vi "file - write list of lines.vi"(7 "read/write control":T1, 10 "list of lines IN":string[](array[string]), 11 "file path":path=path "\\\\rus-one\\newdata/data/Ultrasound/Experiment/ProbeTest/Probe10/Hg1201-6-C185-550Cair-3c-83K/sweep3/9w/3366_a.dat") -> (1 "first line":string, 2 "list of lines OUT":string[](array[string]))   [LabVIEW 2015]
uses:
  file -- read-write control.ctl
  <vilib>/Utility/file.llb/Read From Spreadsheet File (string).vi
  <vilib>/Utility/file.llb/Write To Spreadsheet File (string).vi
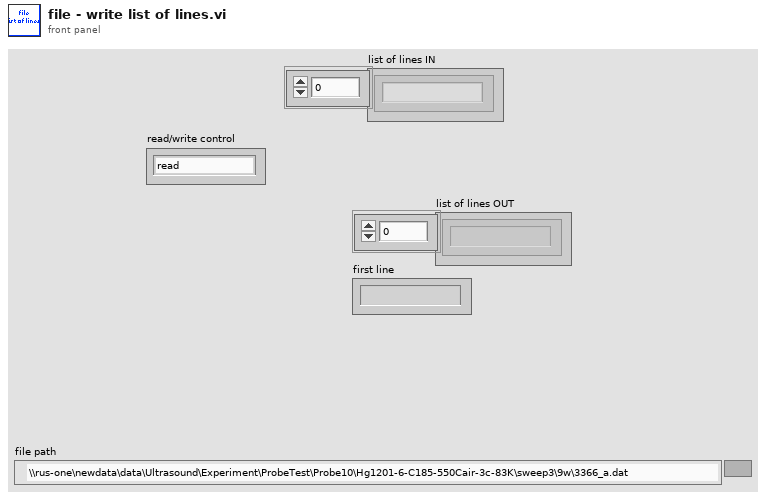
[diagram p1: front panel]
types:
  T1 = typedef "file -- read-write control.ctl" = enum16{"read", "write all", "append one line"}
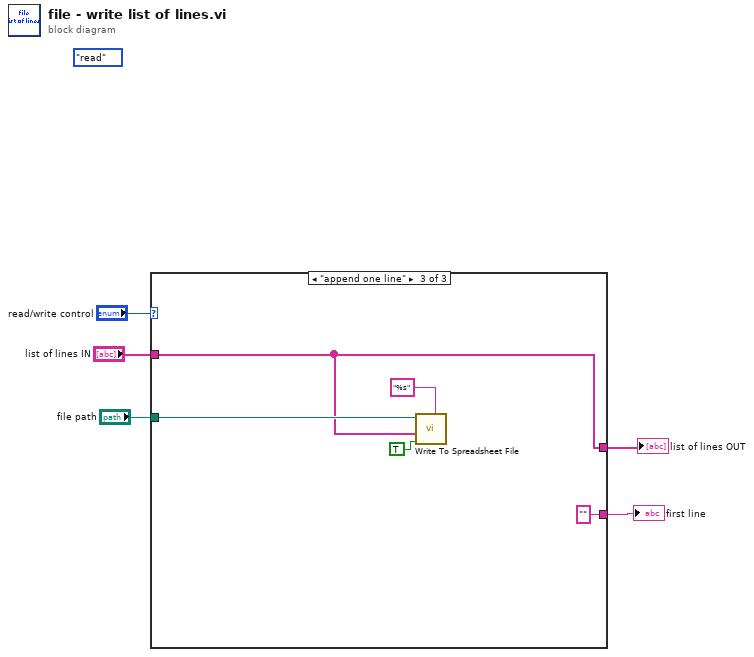
[diagram p0: block diagram]
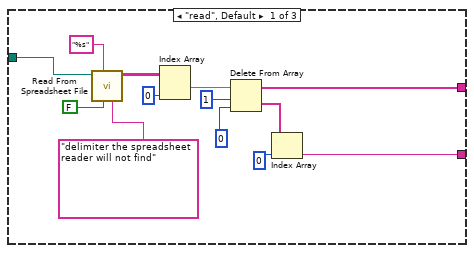
[diagram p2: hidden frame]
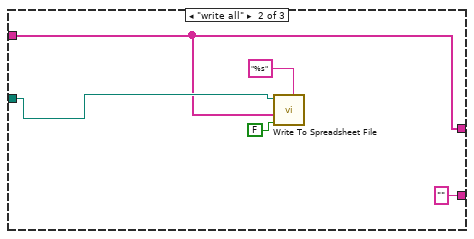
[diagram p3: hidden frame]
diagram:
  (unwired) file_--_read-write_control."read" ("read/write control")
  n1 = case shown="\"append one line\"" "read/write control" {
    tunnel: "file path" -> [w11 w21 w26]
    tunnel: "list of lines IN" -> [_ w20 w24]
    tunnel: [w7 w20 w24] -> w2
    tunnel: [w6 "" ("String") "" ("String")] -> w1
    frame "read", Default {
      n2 = call-poly <vilib>:"Read From Spreadsheet File.vi"("delimiter (\\t)"="delimiter the spreadsheet reader will not find" ("delimiter (\\t)"), "transpose (no:F)"=FALSE ("append to file? (new file:F)"), "format (%s)"="%s", "file path (dialog if empty)"=w11) -> ("all rows"=w16:string[][])  [unwired: 3 in, 4 out]
      n3 = Index Array(array=w16, index (col)=0 ("disabled index (col)")) -> (element=w14:string[])  [unwired: 1 in]
      n4 = Delete From Array(array=w14, length=1, index=0) -> (deleted portion=w9:string[], array with subset deleted=w7:string[])
      n5 = Index Array(array=w9, index=0 ("disabled index (col)")) -> (element=w6:string)
    }
    frame "write all" {
      n6 = call-poly <vilib>:"Write To Spreadsheet File.vi"("format (%s)"="%s", "append to file? (new file:F)"=FALSE, "1D data"=w20, "file path (dialog if empty)"=w21) -> ()  [unwired: 4 in, 1 out]
    }
    frame "append one line" {
      n7 = call-poly <vilib>:"Write To Spreadsheet File.vi"("format (%s)"="%s", "append to file? (new file:F)"=TRUE, "1D data"=w24, "file path (dialog if empty)"=w26) -> ()  [unwired: 4 in, 1 out]
    }
  }
  "list of lines OUT" <- w2
  "first line" <- w1
